vi "Insert.vi"(8 "error in (no error)":errorcluster caption="错误输入（无错误）", 9 "index":i32, 10 "anything":variant caption="任何数据", 11 "ArrayListClass 输入":refnum<class "ArrayListClass.lvclass"> caption="DNL_LabVIEW Object in") -> (0 "error out":errorcluster caption="错误输出", 3 "ArrayListClass 输出":refnum<class "ArrayListClass.lvclass"> caption="DNL_LabVIEW Object out")   [LabVIEW 2012, in "ArrayListClass.lvclass"]
uses:
  ArrayListClass.lvclass
  ArrayListClass.lvclass/ArrayListClass.ctl
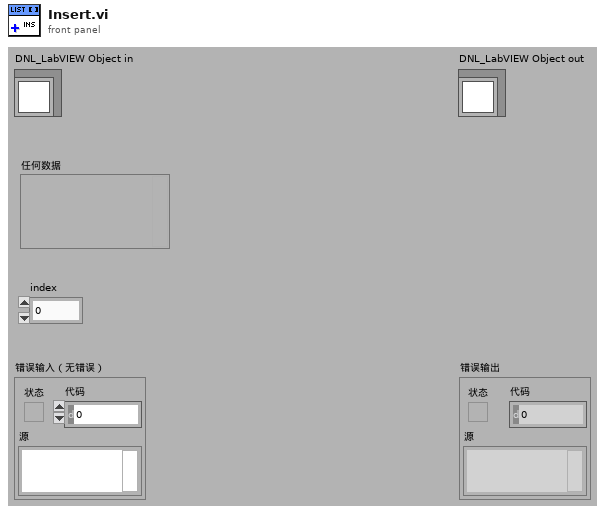
[diagram p1: front panel]
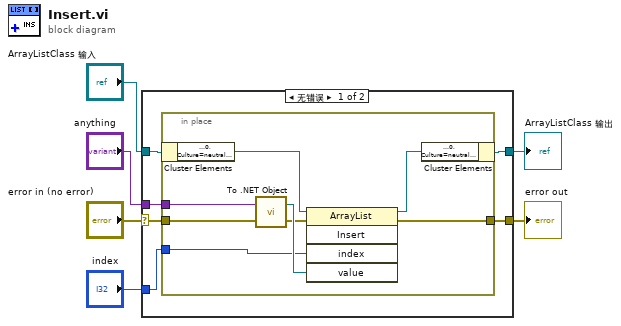
[diagram p0: block diagram]
diagram:
  n1 = case shown="无错误" "error in (no error)" {
    selector: "error in (no error)" -> [w9 w22]
    tunnel: [w8 w22] -> w5
    tunnel: [w10 w21] -> w3
    tunnel: "ArrayListClass 输入" -> [w12 w21]
    tunnel: "anything" -> [w11 _]
    tunnel: "index" -> [w7 _]
    frame No Error {
      n2 = in-place {
        in-place-border: w11 -> [w18]
        in-place-border: w9 -> [w16]
        in-place-border: [w17] -> w8
        in-place-border: w7 -> [w13]
        n3 = in-place-cluster #1(w12) -> ("ArrayList"=w20:refnum<k24>)
        n4 = call <vilib>:"To .NET Object.vi"("error in (no error)"=w16, "anything"=w18) -> ("error out"=w14:errorcluster, ".NET object"=w15:refnum<k24>)
        n5 = invoke class="ArrayList" method="Insert"(reference=w20, error in=w14, "index"=w13, "value"=w15) -> (reference out=w19:refnum<k24>, error out=w17:errorcluster)  [unwired: 1 in, 3 out]
        n6 = in-place-cluster #1("ArrayList"=w19) -> (w10:refnum<class "ArrayListClass.lvclass">)
      }
    }
    frame Error {
    }
  }
  "error out" <- w5
  "ArrayListClass 输出" <- w3
